vi "getMirrorPosition.vi"(6 "Delay between send and receive [ms]":i32=100, 8 "error in (no error)":errorcluster, 10 "locationId":i32, 11 "Monochromator in":refnum<class "Monochromator.lvclass">) -> (0 "error out":errorcluster, 2 "position":i32, 3 "Monochromator out":refnum<class "Monochromator.lvclass">)   [LabVIEW 2020, in "horiba.lvlib" / "Monochromator.lvclass"]
doc: "Returns the position of the specified mirror.\n\nparameter description\nindex Integer. Used to identify which mono to control. See mono_list command\nlocationId Integer. Identifies which mirror to get the position from.\n0 = Mirror 1 (Entrance)\n1 = Mirror 2 (Exit)"
uses:
  Monochromator.lvclass
  Monochromator.lvclass/Monochromator.ctl
  d9b87029-586e-44ee-a6e5-d4a5e0edce38.vi
  b59fd1e7-dcda-425c-bd6c-61aafb79e7f4.vi
  GenericDevice/GenericDevice.lvclass
  MirrorPosition.ctl
  2283113d-39d5-42fa-820e-b0e09e745b74.vi
  <vilib>/JDP Science/JSONtext/JSONtext.lvlib
panel:
  # "Connector Pane"
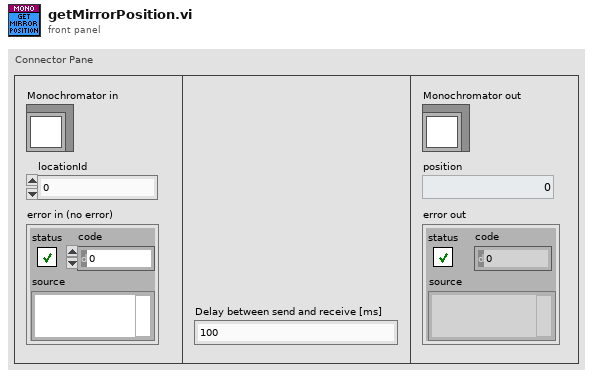
[diagram p1: front panel]
types:
  T1 = typedef "horiba.lvlib/Monochromator.lvclass/MirrorPosition.ctl" = cluster{"position":i32}
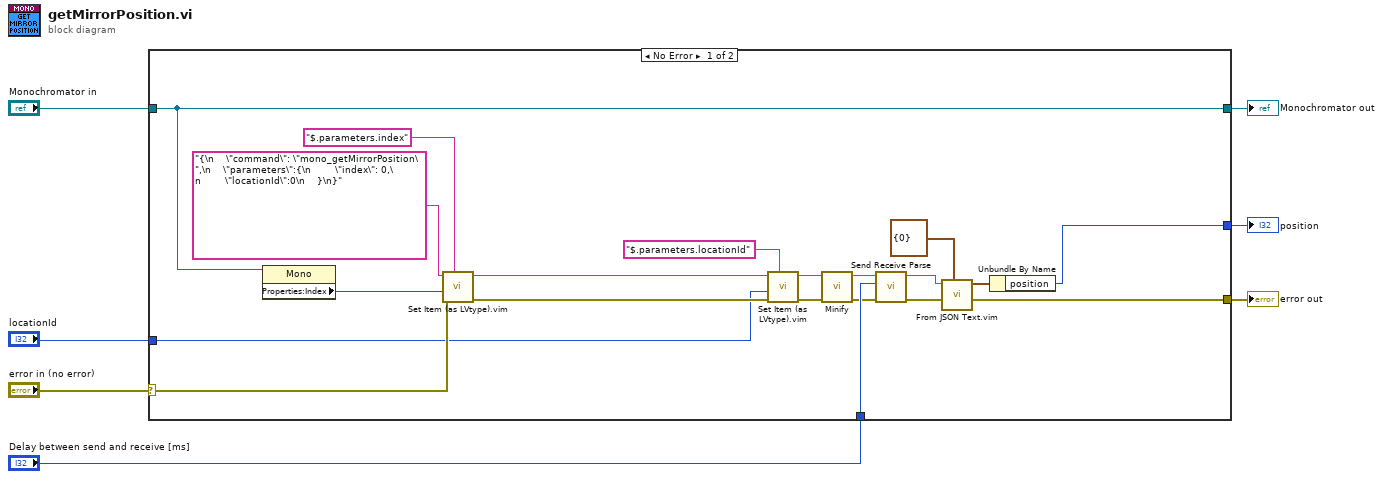
[diagram p0: block diagram]
diagram:
  n1 = case shown="No Error" "error in (no error)" {
    selector: "error in (no error)" -> [w16 w29]
    tunnel: [w26 w29] -> w6
    tunnel: [w17 w28] -> w4
    tunnel: "Monochromator in" -> [w17 w28]
    tunnel: "Delay between send and receive [ms]" -> [w13 _]
    tunnel: "locationId" -> [w12 _]
    tunnel: [w11 _] -> w1
    frame No Error {
      n2 = property class="Mono"(reference=w17) -> ("Properties:Index"=w20:i32)  [unwired: 1 in, 2 out]
      n3 = call "Set Item (as LVtype).vim"("$Path or Item Name"="$.parameters.index", "error in (no error)"=w16, "Anything"=w20, "JSON"="{\n    \"command\": \"mono_getMirrorPosition\",\n    \"parameters\":{\n        \"index\": 0,\n        \"locationId\":0\n    }\n}") -> ("error out"=w15:errorcluster, "<JSON>"=w14:string)  [unwired: 4 in, 1 out]
      n4 = call "Set Item (as LVtype).vim"("$Path or Item Name"="$.parameters.locationId", "error in (no error)"=w15, "Anything"=w12, "JSON"=w14) -> ("error out"=w25:errorcluster, "<JSON>"=w9:string)  [unwired: 4 in, 1 out]
      n5 = call <vilib>:"Minify.vi"("error in (no error)"=w25, "JSON"=w9) -> ("error out"=w10:errorcluster, "<JSON>"=w8:string)  [unwired: 7 in, 1 out]
      n6 = call "Send Receive Parse.vi"("error in"=w10, "Delay between send and receive [ms]"=w13, "<JSON>"=w8) -> ("error out"=w23:errorcluster, "results-JSON string"=w24:string)  [unwired: 6 in, 1 out]
      n7 = call "From JSON Text.vim"("Data Type and Default Value"=T1 {"position"=0} ("Mirror Orientation"), "error in (no error)"=w23, "JSON"=w24) -> ("error out"=w26:errorcluster, "Data out"=w22:T1)  [unwired: 7 in]
      n8 = Unbundle By Name(w22) -> ("position"=w11:i32)
    }
    frame Error {
    }
  }
  "error out" <- w6
  "Monochromator out" <- w4
  "position" <- w1
